vi "Parse Navigation Commands.vi"(8 "error in":errorcluster, 11 "Input":string) -> (0 "error out":errorcluster, 3 "Commands":T1[](array[typedef]))   [LabVIEW 2020, in "Advent of Code.lvlib"]
uses:
  Advent of Code.lvlib
  Navigation Command.ctl
  Navigation Directions.ctl
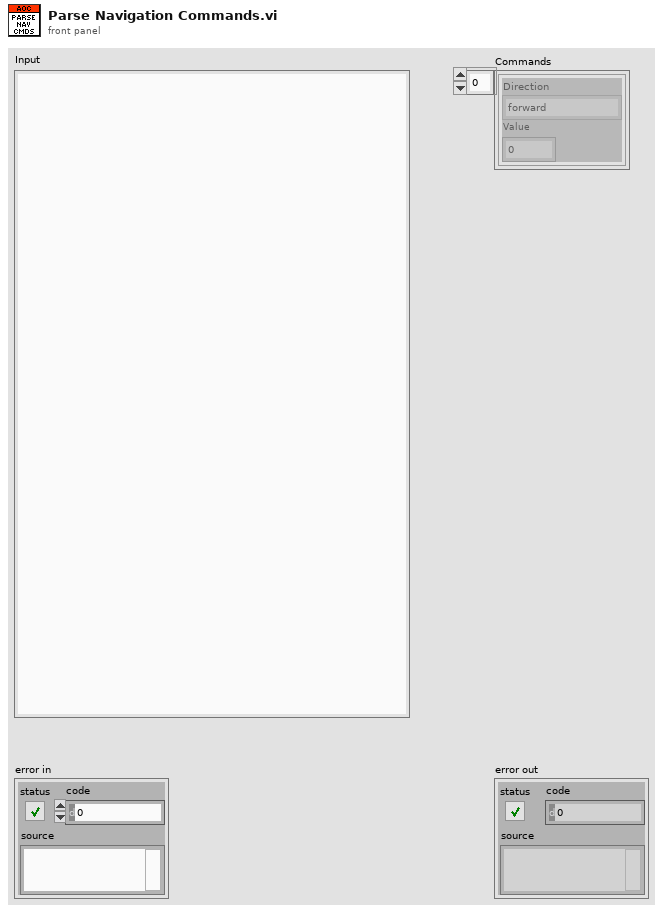
[diagram p1: front panel]
types:
  T1 = typedef "Advent of Code.lvlib/Navigation Command.ctl" = cluster{"Direction":T2, "Value":i32}
  T2 = typedef "Advent of Code.lvlib/Navigation Directions.ctl" = enum16{"forward", "down", "up"}
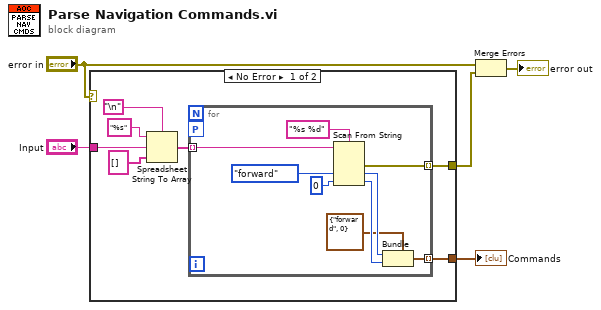
[diagram p0: block diagram]
diagram:
  n1 = case shown="No Error" "error in" {
    tunnel: "Input" -> [w12 _]
    tunnel: [w7 _] -> w4
    tunnel: [w6 _] -> w3
    frame No Error {
      n2 = Spreadsheet String To Array(delimiter (Tab)="\n", format string="%s", spreadsheet string=w12, array type (2D Dbl)=string[] []) -> (array=w9:string[])
      n3 = for {
        tunnel: w9 -> [w21] mode=indexing
        tunnel: [w17] -> w6 mode=indexing
        tunnel: [w14] -> w7 mode=indexing
        workers-P: _ -> [_]
        n4 = Scan From String(format string="%s %d", input string=w21, default 1=Navigation_Directions."forward" ("Navigation Direction"), default 2=0 ("default value 2")) -> (error out=w17:errorcluster, output 1=w16:T2, output 2=w15:i32)  [unwired: 2 in, 2 out]
        n5 = Bundle(cluster=T1 {"Direction"=enum."forward", "Value"=0} ("Navigation Command"), "Direction"=w16, "Value"=w15) -> (w14:T1)
      }
    }
    frame Error {
    }
  }
  "Commands" <- w4
  n6 = Merge Errors("error in", w3) -> (→"error out":errorcluster)
